vi "Core Action.vi"(8 "error in (no error)":errorcluster, 10 "SECS-II Class":refnum<class "SECS-II Class.lvclass">, 11 "28-Remote Control in":refnum<class "28-Remote Control.lvclass">) -> (0 "error out":errorcluster, 2 "SECS-II Class Out":refnum<class "SECS-II Class.lvclass">, 3 "28-Remote Control out":refnum<class "28-Remote Control.lvclass">)   [LabVIEW 2020, in "SECS Scenarios.lvlib" / "28-Remote Control.lvclass"]
uses:
  28-Remote Control.lvclass
  D:/Dropbox/SECS/SECS_GEM v1.1.0/Com/SECS Scenarios/Scenarios Class/Scenarios Class.lvclass
  SECS Communication/SECS-II Class/SECS-II Class.lvclass
  SECS Communication/S2 Message Class/S2 Message Class.lvclass
  D:/Dropbox/SECS/SECS_GEM v1.1.0/Com/SECS Communication/SECS-II Class/SECS-II Class.lvclass
  Remote Command.ctl
  Scenarios Class/Reply State.ctl
  Scenarios Class/Scenarios Class.lvclass/Scenarios Class.ctl
  SECS Communication/S2 Message Class/S2F42.ctl
  Scenarios Class/Write Reply State.vi
  Scenarios Class/Read HSMS Class.vi
  SECS Communication/HSMS Class/HSMS Class.lvclass
  <vilib>/Utility/Data Type/NI_Data Type.lvlib
  Scenarios Class/Scenarios Class.lvclass
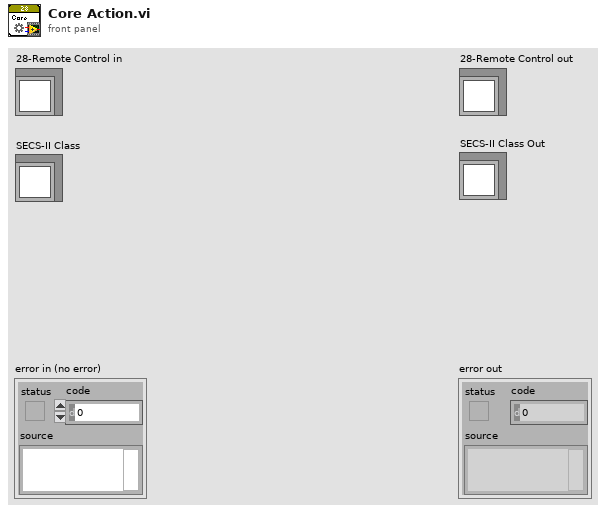
[diagram p1: front panel]
types:
  T1 = typedef "SECS Scenarios.lvlib/28-Remote Control.lvclass/Remote Command.ctl" = enum16{"PP-SELECT", "START", "STOP", "LOCAL", "REMOTE"}
  T2 = typedef "SECS Communication.lvlib/S2 Message Class.lvclass/S2F41.ctl" = cluster{"RCMD":string, "Parameter":cluster{"CPNAME":string, "CPVAL":string}[]}
  T3 = typedef "SECS Scenarios.lvlib/Scenarios Class.lvclass/Reply State.ctl" = enum16{"OK", "Illegal Data", "Unknown Stream", "Unknown Function", "Off-Line", "T3 Timeout", "Inner-Timeout"}
  T4 = cluster{"CPNAME":string, "CPACK":enum8{"unknown CPNAME", "illegal value for CPVAL", "illegal format for CPVAL"}}
  T5 = typedef "SECS Communication.lvlib/S2 Message Class.lvclass/S2F42.ctl" = cluster{"HCACK":enum8{"ok, completed", "invalid command", "cannot do now", "parameter error", "initiated for asynchronous completion", "rejected, already in desired condition", "invalid object"}, "Parameter ":cluster{"CPNAME":string, "CPACK":enum8{"unknown CPNAME", "illegal value for CPVAL", "illegal format for CPVAL"}}[]}
  T6 = enum8{"ok, completed", "invalid command", "cannot do now", "parameter error", "initiated for asynchronous completion", "rejected, already in desired condition", "invalid object"}
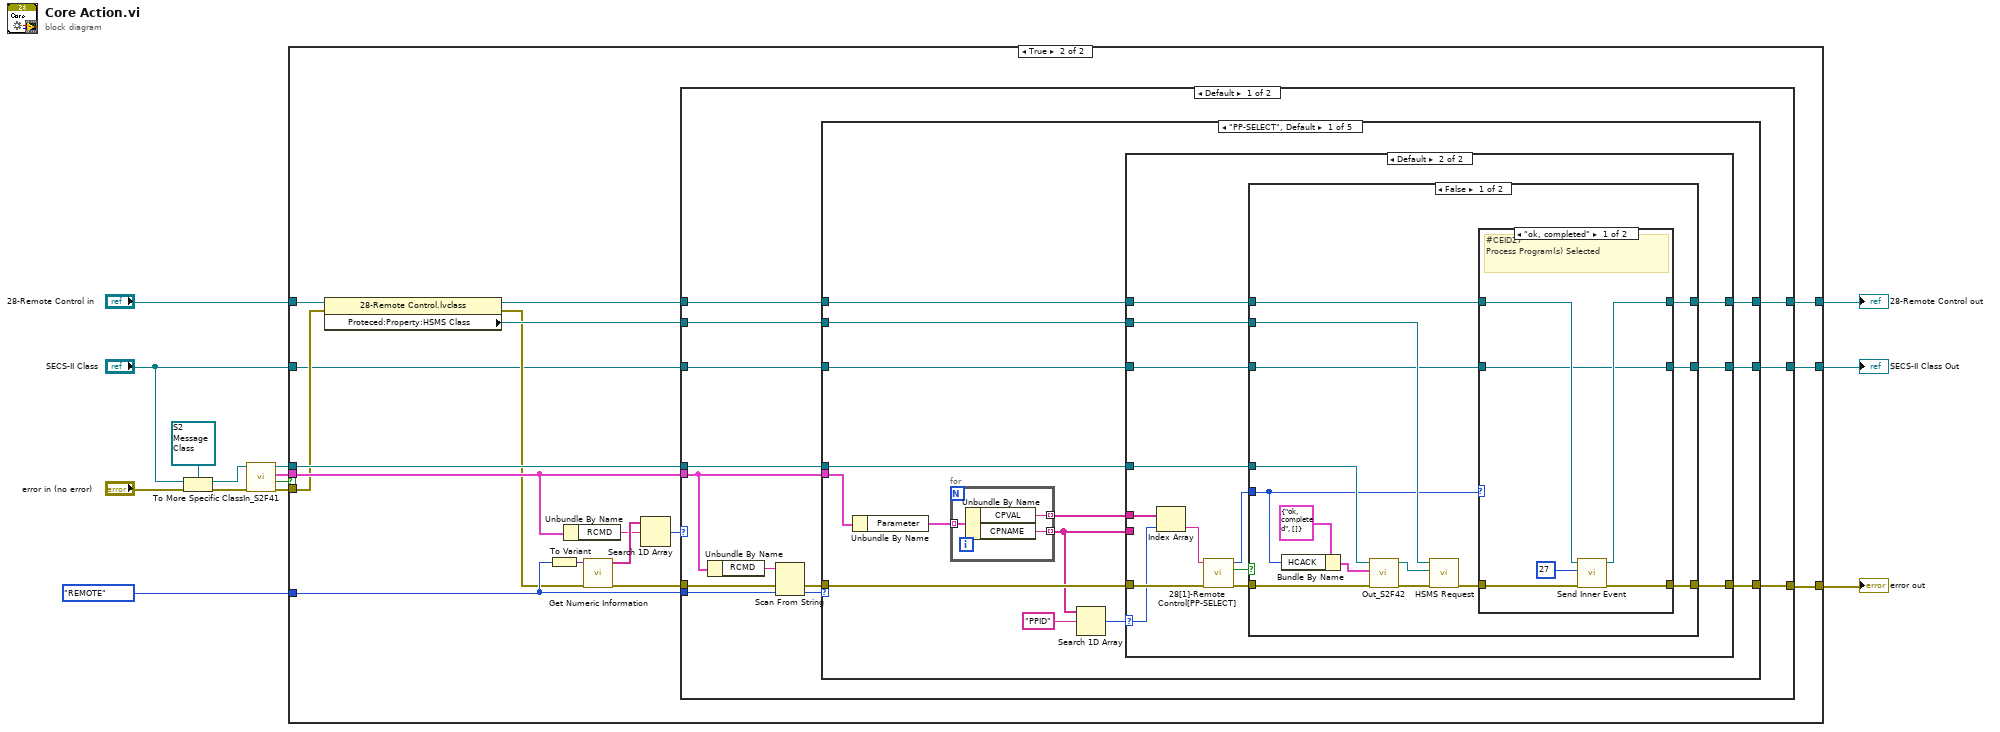
[diagram p0: block diagram]
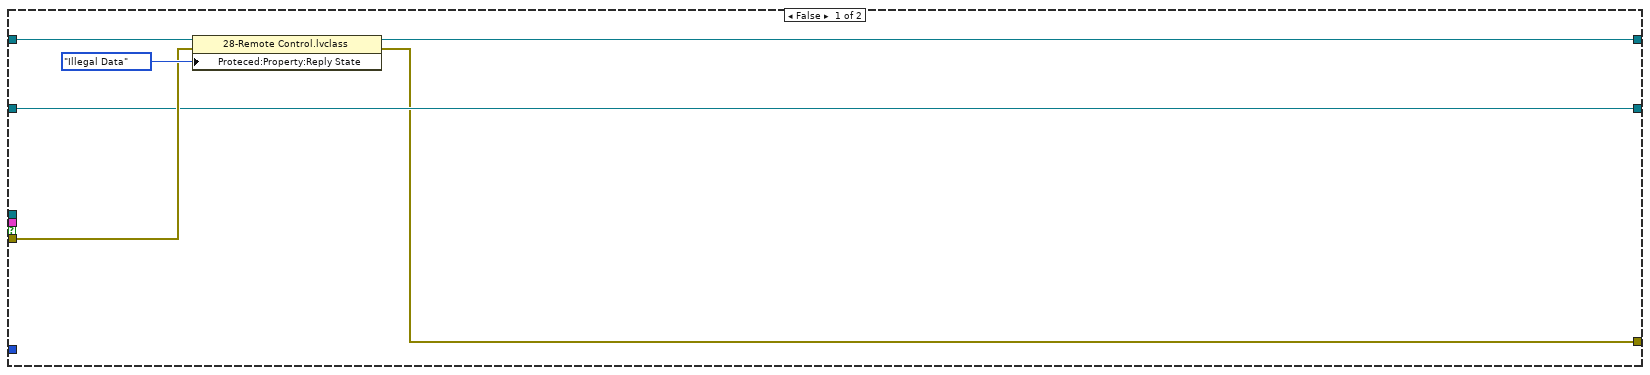
[diagram p2: hidden frame]
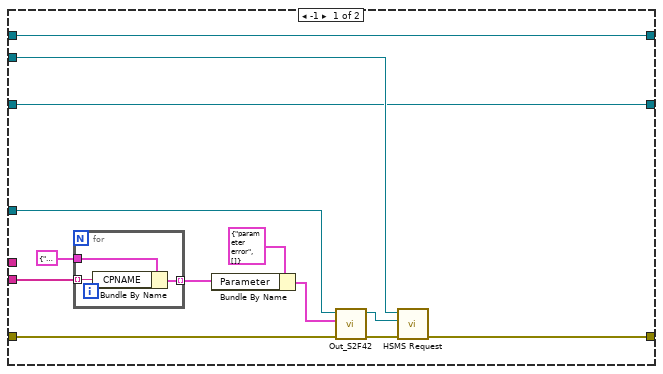
[diagram p3: hidden frame]
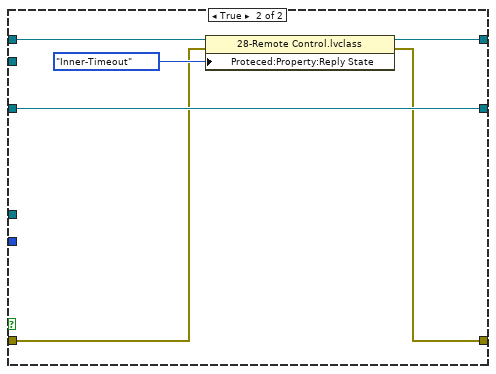
[diagram p5: hidden frame]
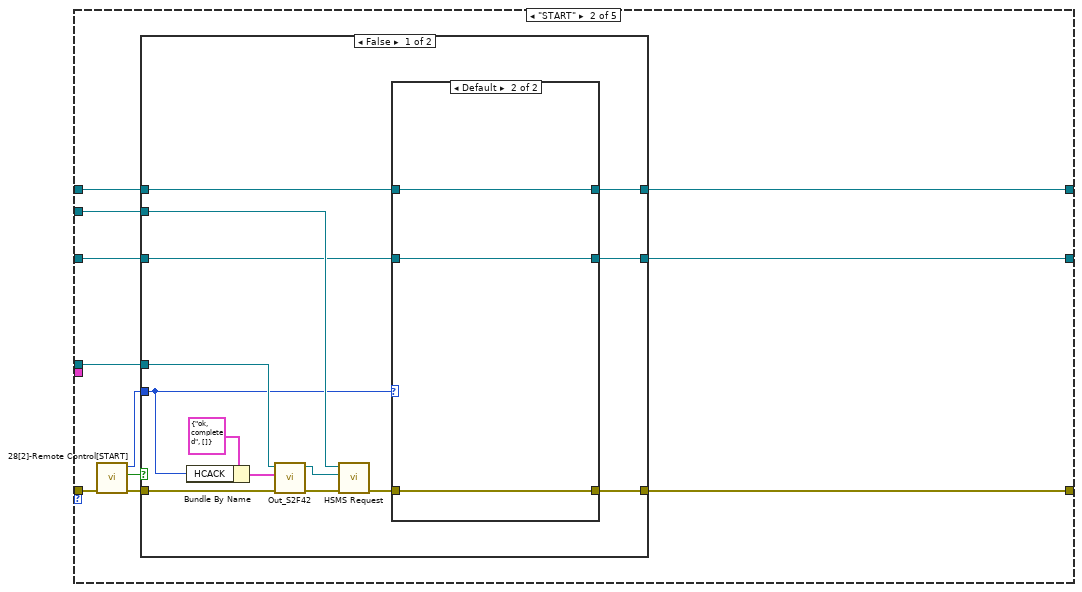
[diagram p6: hidden frame]
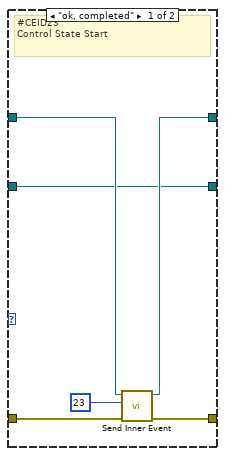
[diagram p7: hidden frame]
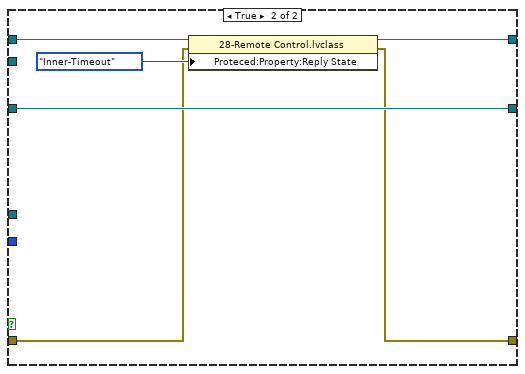
[diagram p8: hidden frame]
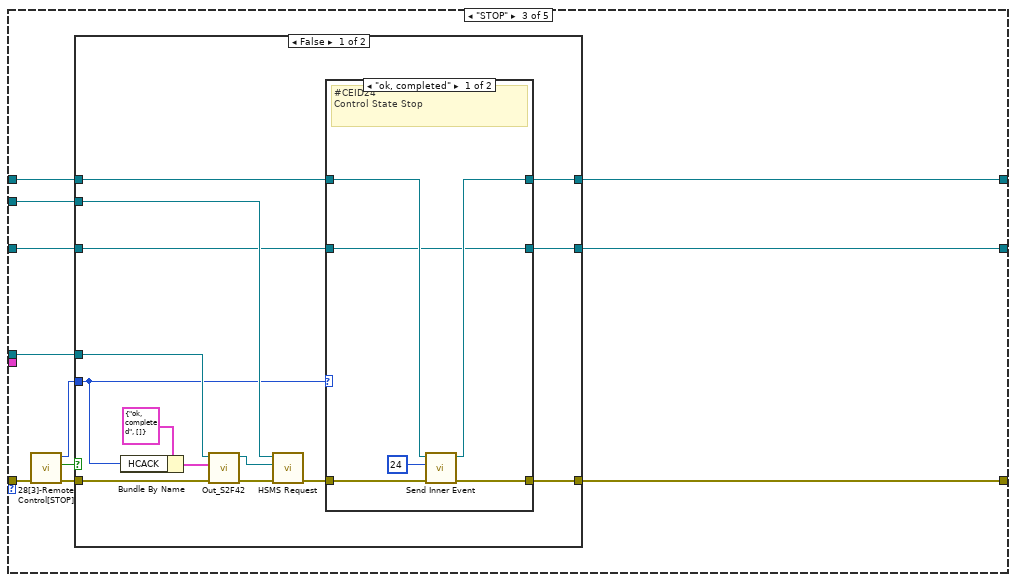
[diagram p9: hidden frame]
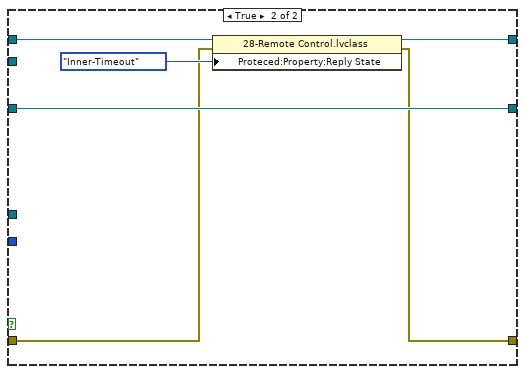
[diagram p11: hidden frame]
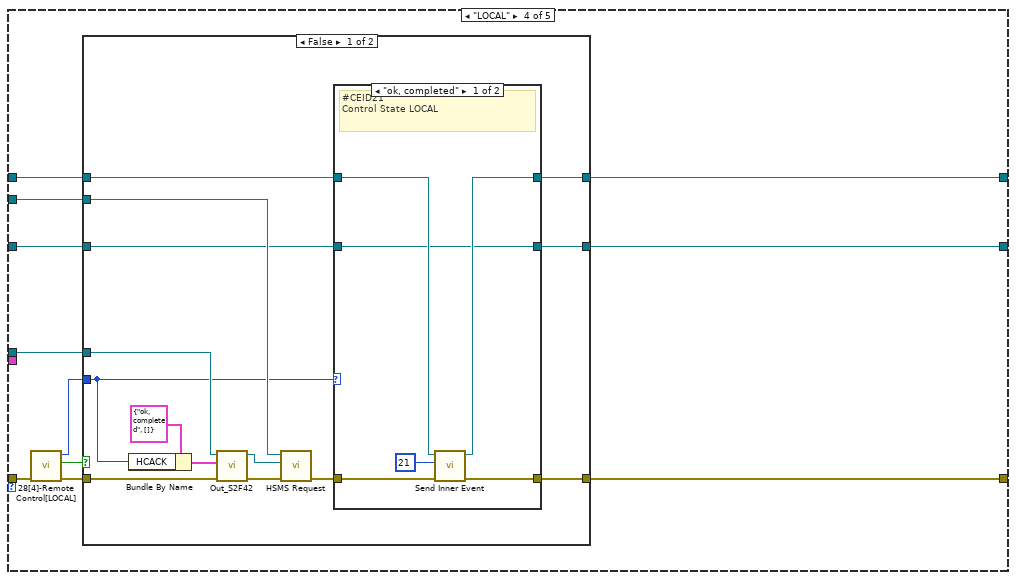
[diagram p12: hidden frame]
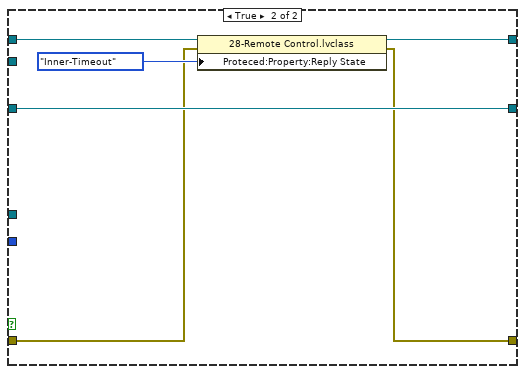
[diagram p14: hidden frame]
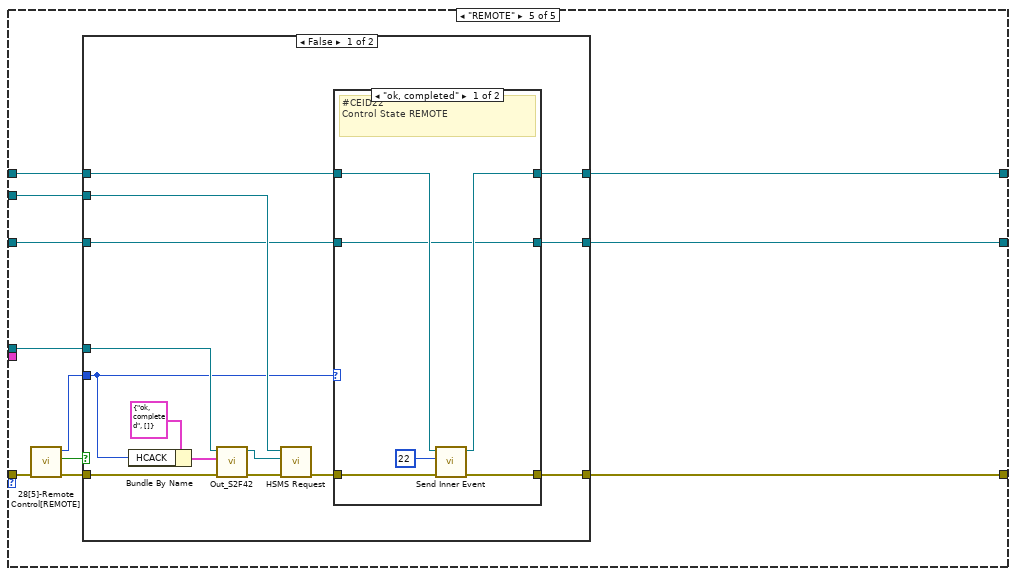
[diagram p15: hidden frame]
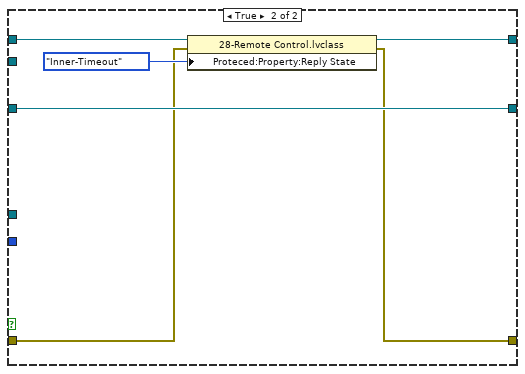
[diagram p17: hidden frame]
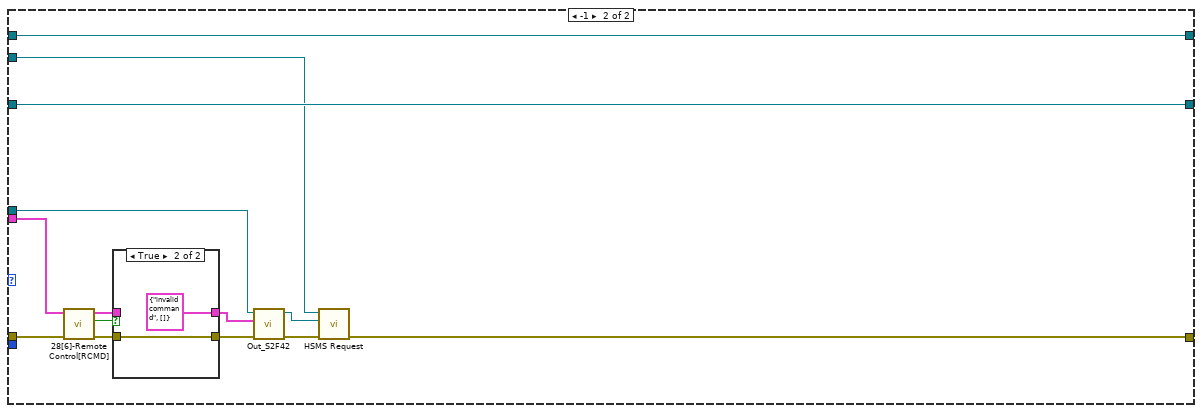
[diagram p18: hidden frame]
diagram:
  n1 = To More Specific Class(target class=refnum<class "S2 Message Class.lvclass"> refnum ("SECS Communication.lvlib:S2 Message Class.lvclass"), reference="SECS-II Class", error in="error in (no error)") -> (specific class reference=w13:refnum<class "S2 Message Class.lvclass">, error out=w14:errorcluster)
  n2 = call "In_S2F41.vi"("error in (no error)"=w14, "S2 Message Class in"=w13) -> ("error out"=w6:errorcluster, "OK?"=w1:bool, "S2F41"=w9:T2, "S2 Message Class out"=w12:refnum<class "S2 Message Class.lvclass">)  [unwired: 6 in]
  n3 = case shown="True" w1 {
    tunnel: w12 -> [_ w37]
    tunnel: w9 -> [_ w31]
    tunnel: Remote_Command."REMOTE" ("Remote Command") -> [_ w30]
    tunnel: "28-Remote Control in" -> [w20 w29]
    tunnel: w6 -> [w18 w27]
    tunnel: [w17 w24] -> w5
    tunnel: [w15 w23] -> w4
    tunnel: "SECS-II Class" -> [w16 w22]
    tunnel: [w16 w21] -> w2
    frame False {
      n4 = property class="28-Remote Control.lvclass"(reference=w20, error in=w18, "Proteced:Property:Reply State"=Reply_State."Illegal Data" ("Reply State")) -> (reference out=w17:refnum<class "28-Remote Control.lvclass">, error out=w15:errorcluster)
    }
    frame True {
      n5 = property class="28-Remote Control.lvclass"(reference=w29, error in=w27) -> (reference out=w28:refnum<class "28-Remote Control.lvclass">, error out=w25:errorcluster, "Proteced:Property:HSMS Class"=w26:refnum<class "HSMS Class.lvclass">)
      n6 = To Variant(anything=w30) -> (Variant=w36:variant)
      n7 = Unbundle By Name(w31) -> ("RCMD"=w34:string)
      n8 = call <vilib>:"Get Numeric Information.vi"("error in (no error)"=w25, "variant"=w36) -> ("error out"=w32:errorcluster, "enum names"=w35:string[])  [unwired: 6 in, 2 out]
      n9 = Search 1D Array(1D array=w35, element=w34) -> (index of element=w33:i32)  [unwired: 1 in]
      n10 = case shown="Default" w33 {
        tunnel: w28 -> [w44 w288]
        tunnel: w37 -> [w45 w291]
        tunnel: [w42 w287] -> w23
        tunnel: w32 -> [w50 w300]
        tunnel: w31 -> [w43 w299]
        tunnel: w30 -> [w48 _]
        tunnel: w26 -> [w41 w289]
        tunnel: [w40 w288] -> w24
        tunnel: w22 -> [w39 w290]
        tunnel: [w38 w290] -> w21
        frame Default {
          n11 = Unbundle By Name(w43) -> ("RCMD"=w49:string)
          n12 = Scan From String(input string=w49, error in=w50, default 1=w48) -> (error out=w46:errorcluster, output 1=w47:T1)  [unwired: 2 in, 2 out]
          n13 = case shown="\"PP-SELECT\", Default" w47 {
            tunnel: w46 -> [w64 w137 w177 w217 w257]
            tunnel: w45 -> [w59 w133 w173 w213 w253]
            tunnel: w44 -> [w58 w131 w171 w211 w251]
            tunnel: w43 -> [w63 _ _ _ _]
            tunnel: [w57 w129 w169 w209 w249] -> w42
            tunnel: w41 -> [w56 w132 w172 w212 w252]
            tunnel: [w55 w130 w170 w210 w250] -> w40
            tunnel: w39 -> [w52 w128 w168 w208 w248]
            tunnel: [w51 w127 w167 w207 w247] -> w38
            frame "PP-SELECT", Default {
              n14 = Unbundle By Name(w63) -> ("Parameter"=w61:cluster{"CPNAME":string, "CPVAL":string}[])
              n15 = for {
                tunnel: w61 -> [w126] mode=indexing
                tunnel: [w125] -> w53 mode=indexing
                tunnel: [w124] -> w54 mode=indexing
                n16 = Unbundle By Name(w126) -> ("CPVAL"=w124:string, "CPNAME"=w125:string)
              }
              n17 = Search 1D Array(1D array=w53, element="PPID") -> (index of element=w60:i32)  [unwired: 1 in]
              n18 = case shown="Default" w60 {
                selector: w60 -> [_ w93]
                tunnel: w64 -> [w71 w94]
                tunnel: w59 -> [w69 w89]
                tunnel: w58 -> [w67 w88]
                tunnel: [w66 w87] -> w57
                tunnel: w56 -> [w68 w86]
                tunnel: [w67 w85] -> w55
                tunnel: w54 -> [_ w84]
                tunnel: w53 -> [w74 _]
                tunnel: w52 -> [w65 w82]
                tunnel: [w65 w81] -> w51
                frame -1 {
                  n19 = for {
                    tunnel: w74 -> [w80] mode=indexing
                    tunnel: T4 {"CPNAME"="", "CPACK"=enum."unknown CPNAME"} ("Parameter") -> [w79]
                    tunnel: [w78] -> w72 mode=indexing
                    n20 = Bundle By Name(cluster=w79, "CPNAME"=w80) -> (w78:T4)
                  }
                  n21 = Bundle By Name(cluster=T5 {"HCACK"=enum."parameter error", "Parameter "=[]} ("S2F42"), "Parameter"=w72) -> (w70:T5)
                  n22 = call "Out_S2F42.vi"("error in (no error)"=w71, "S2F42"=w70, "S2 Message Class in"=w69) -> ("error out"=w76:errorcluster, "S2 Message Class out"=w75:refnum<class "S2 Message Class.lvclass">)  [unwired: 7 in]
                  n23 = call "HSMS Request.vi"("error in (no error)"=w76, "SECS-II Class In"=w75, "HSMS Class in"=w68) -> ("error out"=w66:errorcluster)  [unwired: 7 in, 1 out]
                }
                frame Default {
                  n24 = Index Array(array=w84, index=w93) -> (element=w83:string)
                  n25 = call "28[1]-Remote Control[PP-SELECT].vi"("error in (no error)"=w94, "PPID"=w83) -> ("error out"=w92:errorcluster, "Timeout?"=w91:bool, "HCACK"=w90:T6)  [unwired: 7 in]
                  n26 = case shown="False" w91 {
                    tunnel: w92 -> [w108 w119]
                    tunnel: w90 -> [w101 _]
                    tunnel: w89 -> [w105 _]
                    tunnel: w88 -> [w98 w121]
                    tunnel: [w99 w118] -> w87
                    tunnel: w86 -> [w102 _]
                    tunnel: [w97 w120] -> w85
                    tunnel: w82 -> [w95 w123]
                    tunnel: [w96 w123] -> w81
                    frame False {
                      n27 = Bundle By Name(cluster=T5 {"HCACK"=enum."ok, completed", "Parameter "=[]} ("S2F42"), "HCACK"=w101) -> (w106:T5)
                      n28 = call "Out_S2F42.vi"("error in (no error)"=w108, "S2F42"=w106, "S2 Message Class in"=w105) -> ("error out"=w104:errorcluster, "S2 Message Class out"=w103:refnum<class "S2 Message Class.lvclass">)  [unwired: 7 in]
                      n29 = call "HSMS Request.vi"("error in (no error)"=w104, "SECS-II Class In"=w103, "HSMS Class in"=w102) -> ("error out"=w100:errorcluster)  [unwired: 7 in, 1 out]
                      n30 = case shown="\"ok, completed\"" w101 {
                        tunnel: w100 -> [w114 w117]
                        tunnel: [w110 w117] -> w99
                        tunnel: w98 -> [w112 w115]
                        tunnel: [w111 w115] -> w97
                        tunnel: [w109 w116] -> w96
                        tunnel: w95 -> [w109 w116]
                        frame "ok, completed" {
                          # "#CEID27\nProcess Program(s) Selected"
                          n31 = call "Send Inner Event.vi"("error in (no error)"=w114, "CEID"=u32 27, "Scenarios Class in"=w112) -> ("error out"=w110:errorcluster, "Scenarios Class out"=w111:refnum<class "28-Remote Control.lvclass">)  [unwired: 7 in]
                        }
                        frame Default {
                        }
                      }
                    }
                    frame True {
                      n32 = property class="28-Remote Control.lvclass"(reference=w121, error in=w119, "Proteced:Property:Reply State"=Reply_State."Inner-Timeout" ("Reply State")) -> (reference out=w120:refnum<class "28-Remote Control.lvclass">, error out=w118:errorcluster)
                    }
                  }
                }
              }
            }
            frame "START" {
              n33 = call "28[2]-Remote Control[START].vi"("error in (no error)"=w137) -> ("error out"=w136:errorcluster, "Timeout?"=w135:bool, "HCACK"=w134:T6)  [unwired: 8 in]
              n34 = case shown="False" w135 {
                tunnel: w136 -> [w149 w162]
                tunnel: w134 -> [w143 _]
                tunnel: w133 -> [w146 _]
                tunnel: w132 -> [w145 _]
                tunnel: w131 -> [w141 w164]
                tunnel: [w140 w163] -> w130
                tunnel: [w142 w161] -> w129
                tunnel: w128 -> [w139 w166]
                tunnel: [w138 w166] -> w127
                frame False {
                  n35 = Bundle By Name(cluster=T5 {"HCACK"=enum."ok, completed", "Parameter "=[]} ("S2F42"), "HCACK"=w143) -> (w148:T5)
                  n36 = call "Out_S2F42.vi"("error in (no error)"=w149, "S2F42"=w148, "S2 Message Class in"=w146) -> ("error out"=w151:errorcluster, "S2 Message Class out"=w150:refnum<class "S2 Message Class.lvclass">)  [unwired: 7 in]
                  n37 = call "HSMS Request.vi"("error in (no error)"=w151, "SECS-II Class In"=w150, "HSMS Class in"=w145) -> ("error out"=w144:errorcluster)  [unwired: 7 in, 1 out]
                  n38 = case shown="Default" w143 {
                    tunnel: w144 -> [w157 w160]
                    tunnel: [w156 w160] -> w142
                    tunnel: w141 -> [w154 w159]
                    tunnel: [w153 w159] -> w140
                    tunnel: w139 -> [w152 w158]
                    tunnel: [w152 w158] -> w138
                    frame "ok, completed" {
                      # "#CEID23\nControl State Start"
                      n39 = call "Send Inner Event.vi"("error in (no error)"=w157, "CEID"=u32 23, "Scenarios Class in"=w154) -> ("error out"=w156:errorcluster, "Scenarios Class out"=w153:refnum<class "28-Remote Control.lvclass">)  [unwired: 7 in]
                    }
                    frame Default {
                    }
                  }
                }
                frame True {
                  n40 = property class="28-Remote Control.lvclass"(reference=w164, error in=w162, "Proteced:Property:Reply State"=Reply_State."Inner-Timeout" ("Reply State")) -> (reference out=w163:refnum<class "28-Remote Control.lvclass">, error out=w161:errorcluster)
                }
              }
            }
            frame "STOP" {
              n41 = call "28[3]-Remote Control[STOP].vi"("error in (no error)"=w177) -> ("error out"=w176:errorcluster, "Timeout?"=w175:bool, "HCACK"=w174:T6)  [unwired: 8 in]
              n42 = case shown="False" w175 {
                tunnel: w176 -> [w189 w202]
                tunnel: w174 -> [w183 _]
                tunnel: w173 -> [w186 _]
                tunnel: w172 -> [w185 _]
                tunnel: w171 -> [w181 w204]
                tunnel: [w180 w203] -> w170
                tunnel: [w182 w201] -> w169
                tunnel: w168 -> [w179 w206]
                tunnel: [w178 w206] -> w167
                frame False {
                  n43 = Bundle By Name(cluster=T5 {"HCACK"=enum."ok, completed", "Parameter "=[]} ("S2F42"), "HCACK"=w183) -> (w188:T5)
                  n44 = call "Out_S2F42.vi"("error in (no error)"=w189, "S2F42"=w188, "S2 Message Class in"=w186) -> ("error out"=w191:errorcluster, "S2 Message Class out"=w190:refnum<class "S2 Message Class.lvclass">)  [unwired: 7 in]
                  n45 = call "HSMS Request.vi"("error in (no error)"=w191, "SECS-II Class In"=w190, "HSMS Class in"=w185) -> ("error out"=w184:errorcluster)  [unwired: 7 in, 1 out]
                  n46 = case shown="\"ok, completed\"" w183 {
                    tunnel: w184 -> [w197 w200]
                    tunnel: [w193 w200] -> w182
                    tunnel: w181 -> [w195 w199]
                    tunnel: [w194 w199] -> w180
                    tunnel: w179 -> [w192 w198]
                    tunnel: [w192 w198] -> w178
                    frame "ok, completed" {
                      # "#CEID24\nControl State Stop"
                      n47 = call "Send Inner Event.vi"("error in (no error)"=w197, "CEID"=u32 24, "Scenarios Class in"=w195) -> ("error out"=w193:errorcluster, "Scenarios Class out"=w194:refnum<class "28-Remote Control.lvclass">)  [unwired: 7 in]
                    }
                    frame Default {
                    }
                  }
                }
                frame True {
                  n48 = property class="28-Remote Control.lvclass"(reference=w204, error in=w202, "Proteced:Property:Reply State"=Reply_State."Inner-Timeout" ("Reply State")) -> (reference out=w203:refnum<class "28-Remote Control.lvclass">, error out=w201:errorcluster)
                }
              }
            }
            frame "LOCAL" {
              n49 = call "28[4]-Remote Control[LOCAL].vi"("error in (no error)"=w217) -> ("error out"=w216:errorcluster, "Timeout?"=w215:bool, "HCACK"=w214:T6)  [unwired: 8 in]
              n50 = case shown="False" w215 {
                tunnel: w216 -> [w229 w243]
                tunnel: w214 -> [w223 _]
                tunnel: w213 -> [w226 _]
                tunnel: w212 -> [w225 _]
                tunnel: w211 -> [w221 w244]
                tunnel: [w220 w242] -> w210
                tunnel: [w222 w241] -> w209
                tunnel: w208 -> [w219 w246]
                tunnel: [w218 w246] -> w207
                frame False {
                  n51 = Bundle By Name(cluster=T5 {"HCACK"=enum."ok, completed", "Parameter "=[]} ("S2F42"), "HCACK"=w223) -> (w228:T5)
                  n52 = call "Out_S2F42.vi"("error in (no error)"=w229, "S2F42"=w228, "S2 Message Class in"=w226) -> ("error out"=w231:errorcluster, "S2 Message Class out"=w230:refnum<class "S2 Message Class.lvclass">)  [unwired: 7 in]
                  n53 = call "HSMS Request.vi"("error in (no error)"=w231, "SECS-II Class In"=w230, "HSMS Class in"=w225) -> ("error out"=w224:errorcluster)  [unwired: 7 in, 1 out]
                  n54 = case shown="\"ok, completed\"" w223 {
                    tunnel: w224 -> [w237 w240]
                    tunnel: [w233 w240] -> w222
                    tunnel: w221 -> [w235 w239]
                    tunnel: [w234 w239] -> w220
                    tunnel: w219 -> [w232 w238]
                    tunnel: [w232 w238] -> w218
                    frame "ok, completed" {
                      # "#CEID21\nControl State LOCAL"
                      n55 = call "Send Inner Event.vi"("error in (no error)"=w237, "CEID"=u32 21, "Scenarios Class in"=w235) -> ("error out"=w233:errorcluster, "Scenarios Class out"=w234:refnum<class "28-Remote Control.lvclass">)  [unwired: 7 in]
                    }
                    frame Default {
                    }
                  }
                }
                frame True {
                  n56 = property class="28-Remote Control.lvclass"(reference=w244, error in=w243, "Proteced:Property:Reply State"=Reply_State."Inner-Timeout" ("Reply State")) -> (reference out=w242:refnum<class "28-Remote Control.lvclass">, error out=w241:errorcluster)
                }
              }
            }
            frame "REMOTE" {
              n57 = call "28[5]-Remote Control[REMOTE].vi"("error in (no error)"=w257) -> ("error out"=w256:errorcluster, "Timeout?"=w255:bool, "HCACK"=w254:T6)  [unwired: 8 in]
              n58 = case shown="False" w255 {
                tunnel: w256 -> [w269 w283]
                tunnel: w254 -> [w263 _]
                tunnel: w253 -> [w266 _]
                tunnel: w252 -> [w265 _]
                tunnel: w251 -> [w261 w284]
                tunnel: [w260 w282] -> w250
                tunnel: [w262 w281] -> w249
                tunnel: w248 -> [w259 w286]
                tunnel: [w258 w286] -> w247
                frame False {
                  n59 = Bundle By Name(cluster=T5 {"HCACK"=enum."ok, completed", "Parameter "=[]} ("S2F42"), "HCACK"=w263) -> (w268:T5)
                  n60 = call "Out_S2F42.vi"("error in (no error)"=w269, "S2F42"=w268, "S2 Message Class in"=w266) -> ("error out"=w271:errorcluster, "S2 Message Class out"=w270:refnum<class "S2 Message Class.lvclass">)  [unwired: 7 in]
                  n61 = call "HSMS Request.vi"("error in (no error)"=w271, "SECS-II Class In"=w270, "HSMS Class in"=w265) -> ("error out"=w264:errorcluster)  [unwired: 7 in, 1 out]
                  n62 = case shown="\"ok, completed\"" w263 {
                    tunnel: w264 -> [w277 w280]
                    tunnel: [w272 w280] -> w262
                    tunnel: w261 -> [w275 w279]
                    tunnel: [w274 w279] -> w260
                    tunnel: w259 -> [w273 w278]
                    tunnel: [w273 w278] -> w258
                    frame "ok, completed" {
                      # "#CEID22\nControl State REMOTE"
                      n63 = call "Send Inner Event.vi"("error in (no error)"=w277, "CEID"=u32 22, "Scenarios Class in"=w275) -> ("error out"=w272:errorcluster, "Scenarios Class out"=w274:refnum<class "28-Remote Control.lvclass">)  [unwired: 7 in]
                    }
                    frame Default {
                    }
                  }
                }
                frame True {
                  n64 = property class="28-Remote Control.lvclass"(reference=w284, error in=w283, "Proteced:Property:Reply State"=Reply_State."Inner-Timeout" ("Reply State")) -> (reference out=w282:refnum<class "28-Remote Control.lvclass">, error out=w281:errorcluster)
                }
              }
            }
          }
        }
        frame -1 {
          n65 = call "28[6]-Remote Control[RCMD].vi"("error in (no error)"=w300, "S2F41"=w299) -> ("error out"=w298:errorcluster, "Timeout?"=w297:bool, "S2F42"=w296:T5)  [unwired: 7 in]
          n66 = case shown="True" w297 {
            tunnel: w298 -> [w301 w304]
            tunnel: w296 -> [w302 _]
            tunnel: [w301 w304] -> w293
            tunnel: [w302 T5 {"HCACK"=enum."invalid command", "Parameter "=[]} ("S2F42")] -> w292
            frame False {
            }
            frame True {
            }
          }
          n67 = call "Out_S2F42.vi"("error in (no error)"=w293, "S2F42"=w292, "S2 Message Class in"=w291) -> ("error out"=w294:errorcluster, "S2 Message Class out"=w295:refnum<class "S2 Message Class.lvclass">)  [unwired: 7 in]
          n68 = call "HSMS Request.vi"("error in (no error)"=w294, "SECS-II Class In"=w295, "HSMS Class in"=w289) -> ("error out"=w287:errorcluster)  [unwired: 7 in, 1 out]
        }
      }
    }
  }
  "error out" <- w4
  "28-Remote Control out" <- w5
  "SECS-II Class Out" <- w2
